vi "GetIDfromName.vi"(9 "name":T1, 11 "meta data":T1[](array[typedef])) -> (1 "found?":bool, 3 "meta ID":u16)   [LabVIEW 2010, in "NI STM.lvlib"]
doc: "This VI looks up the Meta data index using the Meta data name.\n\nCopyright 2015, 2016, 2017 National Instruments Corporation\n\nLicensed under the Apache License, Version 2.0 (the \"License\"); you may not use this file except in compliance with the License.\n\n You may obtain a copy of the License at\n\n http://www.apache.org/licenses/LICENSE-2.0\n\nUnless required by applicable law or agreed to in writing, software distributed under the License is distributed on an \"AS IS\" BASIS, WITHOUT WARRANTIES OR CONDITIONS OF ANY KIND, either express or implied.\n\nSee the License for the specific language governing permissions and limitations under the License."
uses:
  NI STM.lvlib
  MetaDataElement.ctl
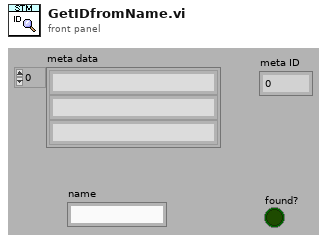
[diagram p1: front panel]
types:
  T1 = typedef "NI STM.lvlib/MetaDataElement.ctl" = string
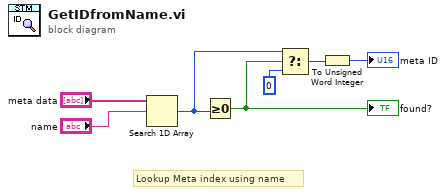
[diagram p0: block diagram]
diagram:
  # "Lookup Meta index using name"
  n1 = Search 1D Array(1D array="meta data", element="name") -> (index of element=w3:i32)  [unwired: 1 in]
  n2 = Greater Or Equal To 0?(x=w3) -> (x >= 0?=w4:bool)
  "found?" <- w4
  n3 = Select(t=w3, s=w4, f=0) -> (s? t:f=w2:i32)
  n4 = To Unsigned Word Integer(number=w2) -> (unsigned 16bit integer=→"meta ID":u16)
